vi "GE 5565PIORC.DMA.Block.Write (DBL).vi"(7 "byte order (big-endian)":T1(ring), 8 "error in (no error)":errorcluster, 9 "data":dbl[](array[numeric]), 10 "Block Descriptor in":T2 {"descriptor params"."data ptr (lower)" format="%.0x"; "descriptor params"."data ptr (upper)" format="%.0x"; "descriptor params"."data size" format="%.0x"; "descriptor params"."next descriptor ptr" format="%.0x"; "descriptor size" format="%08x"; "descriptor ptr (RFM)" format="%08x"; "descriptor ptr (VISA)" format="%08x"}, 11 "GE 5565PIORC in":refnum<class "GE 5565PIORC.lvclass">) -> (0 "error out":errorcluster, 1 "data out":dbl[](array[numeric]), 2 "Block Descriptor out":T2 {"descriptor params"."data ptr (lower)" format="%.0x"; "descriptor params"."data ptr (upper)" format="%.0x"; "descriptor params"."data size" format="%.0x"; "descriptor params"."next descriptor ptr" format="%.0x"; "descriptor size" format="%08x"; "descriptor ptr (RFM)" format="%08x"; "descriptor ptr (VISA)" format="%08x"}, 3 "GE 5565PIORC out":refnum<class "GE 5565PIORC.lvclass">)   [LabVIEW 2020, in "GE 5565PIORC.lvclass"]
doc: "Writes the contents of the <B>data</B> array to the specified <B>Block Descriptor</B>. The number of elements transferred will be either the number of elements in <B>data</B> or a number of elements resulting in a size that is less than or equal to the allocated size of the <B>Block Descriptor</B>, whichever is smaller."
uses:
  GE 5565PIORC.lvclass
  Typedefs/GE 5565PIORC.Typedef.DMA Block Descriptor.ctl
  Typedefs/GE 5565PIORC.Typedef.DMA Block Descriptor Params.ctl
  <vilib>/Instr/_visa.llb/VISA Register Access Address Space.ctl
  GE 5565PIORC.lvclass/GE 5565PIORC.ctl
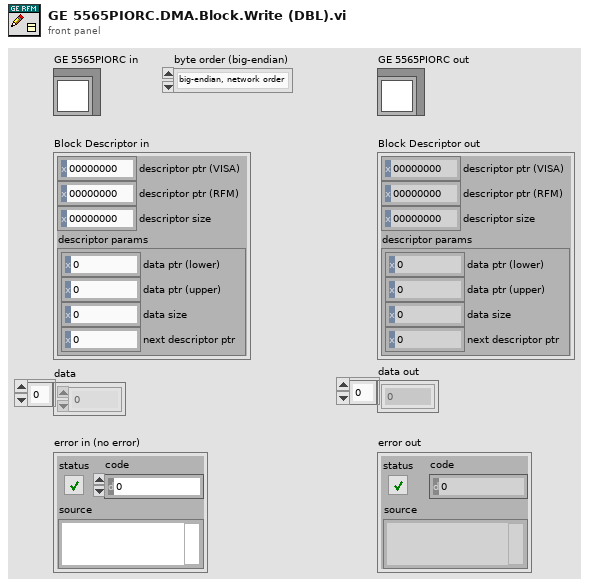
[diagram p1: front panel]
types:
  T1 = enum16{"big-endian, network order", "native, host order", "little-endian"}
  T2 = typedef "GE 5565PIORC.lvclass/GE 5565PIORC.Typedef.DMA Block Descriptor.ctl" = cluster{"descriptor ptr (VISA)":u32, "descriptor ptr (RFM)":u32, "descriptor size":u32, "descriptor params":T3}
  T3 = typedef "GE 5565PIORC.lvclass/GE 5565PIORC.Typedef.DMA Block Descriptor Params.ctl" = cluster{"data ptr (lower)":u32, "data ptr (upper)":u32, "data size":u32, "next descriptor ptr":u32}
  T4 = typedef "VISA Register Access Address Space.ctl" = u16
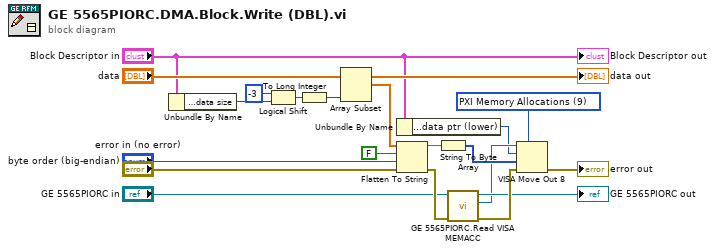
[diagram p0: block diagram]
diagram:
  w13 = T4 9 items=["VXI/VME A16"=1, "VXI/VME A24"=2, "VXI/VME A32"=3, "VXI/VME A64"=4, "PXI Memory Allocations"=9, "PXI Configuration"=10, "PXI BAR0"=11, "PXI BAR1"=12, "PXI BAR2"=13, "PXI BAR3"=14, "PXI BAR4"=15, "PXI BAR5"=16] ("address space")
  n1 = Unbundle By Name("Block Descriptor in") -> ("descriptor params.data size"=w12:u32)
  n2 = Logical Shift(y=i16 -3, x=w12) -> (x << y=w18:u32)
  n3 = To Long Integer(number=w18) -> (32bit integer=w19:i32)
  n4 = Array Subset(array="data", length=w19) -> (w17:dbl[])  [unwired: 1 in]
  n5 = Unbundle By Name("Block Descriptor in") -> ("descriptor params.data ptr (lower)"=w2:u32)
  n6 = Flatten To String(anything=w17, prepend array or string size? (T)=FALSE, byte order (0:big-endian, network order)="byte order (big-endian)", error in (no error)="error in (no error)") -> (data string=w11:string, error out=w7:errorcluster)  [unwired: 1 out]
  n7 = String To Byte Array(string=w11) -> (unsigned byte array=w14:u8[])
  n8 = call "GE 5565PIORC.Read VISA MEMACC.vi"("error in (no error)"=w7, "GE 5565PIORC in"="GE 5565PIORC in") -> ("error out"=w6:errorcluster, "VISA MEMACC"=w3:refnum<visa-resource-name>, "GE 5565PIORC out"=→"GE 5565PIORC out":refnum<class "GE 5565PIORC.lvclass">)  [unwired: 7 in]
  n9 = VISA Move Out 8(7:w13, 8:w6, 9:w14, 10:w2, 11:w3) -> (0:→"error out":errorcluster)  [unwired: 1 out]
  "Block Descriptor out" <- "Block Descriptor in"
  "data out" <- "data"
